vi "_PC_Spectrafilter block_interface_for_sn.vi"(7 "enable":bool, 8 "error in (no error)":errorcluster, 9 "Pane 2":refnum<vi>, 10 "Pane":refnum<vi>, 11 "mouse state":refnum<vi>) -> (0 "error out":errorcluster)   [LabVIEW 2018]
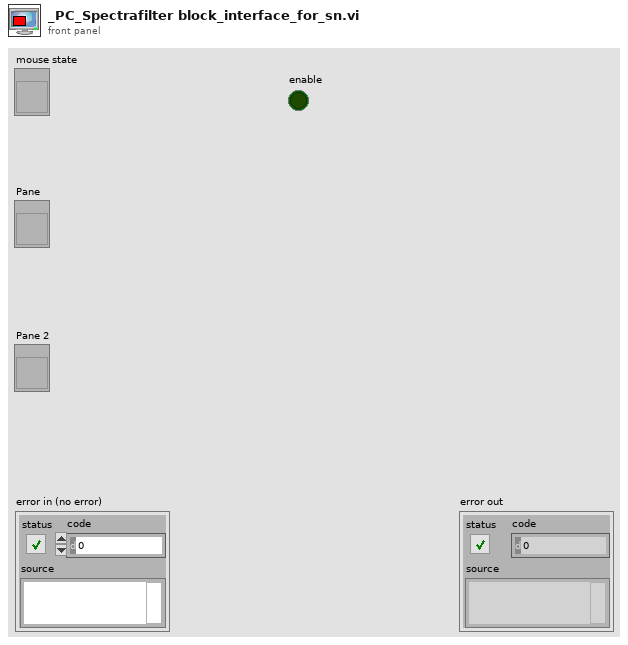
[diagram p1: front panel]
types:
  T1 = enum8{"Enabled", "Disabled", "Disabled and Grayed Out"}
  T2 = enum16{"normal", "select noise", "select signal"}
  T3 = enum16{"normal", "select noise", "select signal", "return"}
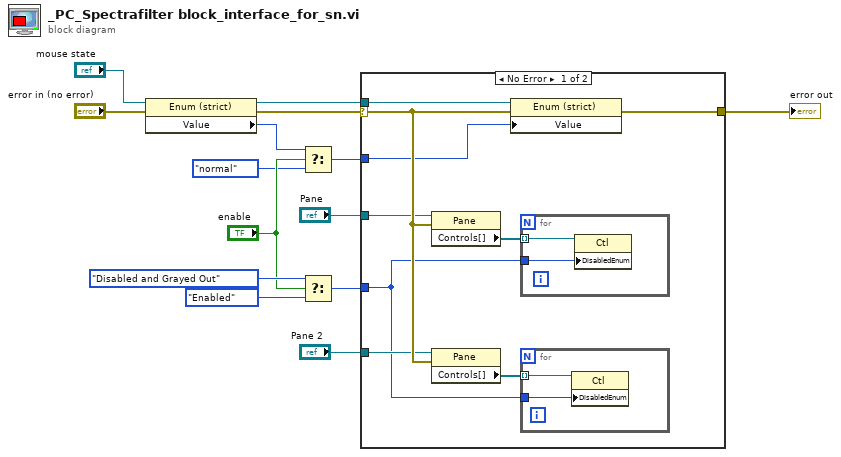
[diagram p0: block diagram]
diagram:
  n1 = property class="Enum (strict)"(reference="mouse state", error in="error in (no error)") -> (reference out=w3:refnum<vi>, error out=w2:errorcluster, "Value"=w1:T3)
  n2 = Select(t=w1, s="enable", f=T2."normal" ("Value")) -> (s? t:f=w8:T3)
  n3 = Select(t=T1."Disabled and Grayed Out" ("Disabled"), s="enable", f=T1."Enabled" ("Disabled")) -> (s? t:f=w7:T1)
  n4 = case shown="No Error" w2 {
    selector: w2 -> [w20 w28]
    tunnel: w3 -> [w21 _]
    tunnel: [w19 w28] -> w14
    tunnel: "Pane" -> [w18 _]
    tunnel: "Pane 2" -> [w17 _]
    tunnel: w8 -> [w16 _]
    tunnel: w7 -> [w15 _]
    frame No Error {
      n5 = property class="Pane"(reference=w18, error in=w20) -> ("Controls[]"=w23:refnum<vi>[])  [unwired: 2 out]
      n6 = property class="Pane"(reference=w17, error in=w20) -> ("Controls[]"=w22:refnum<vi>[])  [unwired: 2 out]
      n7 = property class="Enum (strict)"(reference=w21, error in=w20, "Value"=w16) -> (error out=w19:errorcluster)  [unwired: 1 out]
      n8 = for {
        tunnel: w23 -> [w27] mode=indexing
        tunnel: w15 -> [w26]
        n9 = property class="Ctl"(reference=w27, "DisabledEnum"=w26) -> ()  [unwired: 1 in, 2 out]
      }
      n10 = for {
        tunnel: w22 -> [w25] mode=indexing
        tunnel: w15 -> [w24]
        n11 = property class="Ctl"(reference=w25, "DisabledEnum"=w24) -> ()  [unwired: 1 in, 2 out]
      }
    }
    frame Error {
    }
  }
  "error out" <- w14
